vi "Add Item.vi"(7 "Action":T1, 8 "error in (no error)":errorcluster, 11 "Listbox Refs in":T2 {"Section Ref" format="%.0x"}) -> (0 "error out":errorcluster, 3 "Listbox Refs out":T2 {"Section Ref" format="%.0x"})   [LabVIEW 2015, in "FPGA Addon System Explorer.lvlib"]
uses:
  FPGA Addon System Explorer.lvlib
  Listbox Cluster.ctl
  <vilib>/NI Veristand/Custom Device API/Custom Device Item Ref.ctl
  Channel Type.ctl
  Shared/FG Action.ctl
  <vilib>/NI Veristand/Custom Device API/Custom Device Channel.ctl
  <vilib>/NI Veristand/Custom Device API/Custom Device Channel Type.ctl
  SubModules/FPGA Addon Speciality IO/Source/Types/PWM.Measure.Analog.Settings.ctl
  SubModules/FPGA Addon Speciality IO/Source/Types/PWM.Generate.Digital.Settings.ctl
  SubModules/FPGA Addon Speciality IO/Source/Types/PWM.Generate.Digital.Convert.Settings.ctl
  SubModules/FPGA Addon Speciality IO/Source/Types/WSS.Generate.Digital.Settings.ctl
  SubModules/FPGA Addon Speciality IO/Source/Types/WSS.Generate.Digital.Convert.Settings.ctl
  SubModules/FPGA Addon Speciality IO/Source/Types/WSS.Sensor.Type.ctl
  SubModules/FPGA Addon Speciality IO/Source/Types/Static.Generate.Digital.Settings.ctl
  SubModules/FPGA Addon Speciality IO/Source/Types/Static.Measure.Digital.Settings.ctl
  SubModules/FPGA Addon Speciality IO/Source/Types/Sine.Generate.Settings.ctl
  SubModules/FPGA Addon Speciality IO/Source/Types/Sine.Generate.Convert.Settings.ctl
  SubModules/FPGA Addon Speciality IO/Source/Types/PWM.Measure.Digital.Settings.ctl
  SubModules/FPGA Addon Speciality IO/Source/Types/PWM.Measure.Analog.Result.ctl
  SubModules/FPGA Addon Speciality IO/Source/Types/PWM.Measure.Digital.Result.ctl
  SubModules/FPGA Addon Speciality IO/Source/Types/Static.Measure.Digital.Measurement.ctl
  Shared/Constants.vi
  <vilib>/NI Veristand/Custom Device API/NI VeriStand - Set Item Property.vi
  <vilib>/NI Veristand/Custom Device API/Set Item Property (Variant).vi
  <vilib>/NI Veristand/Custom Device API/NI VeriStand - Get Item Property.vi
  <vilib>/NI Veristand/Custom Device API/Get Item Property (Variant).vi
  <vilib>/NI VeriStand/Custom Device API/Custom Device API.lvlib
  Shared/FPGA Addon Shared.lvlib
  SubModules/FPGA Addon Speciality IO/Source/Speciality FPGA IO.lvlib
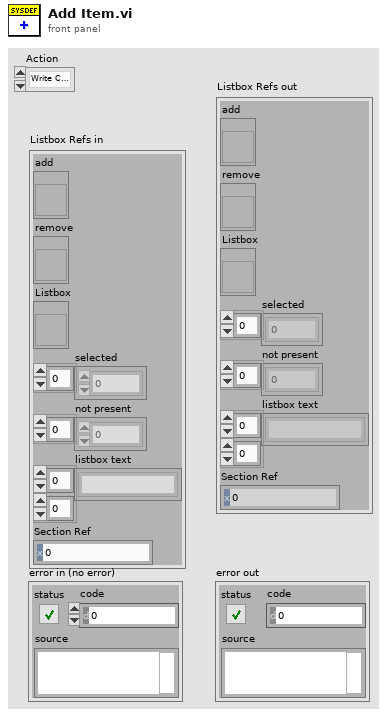
[diagram p1: front panel]
types:
  T1 = typedef "FPGA Addon System Explorer.lvlib/Channel Type.ctl" = enum16{"Write Channel", "Read Channel", "Write Waveform", "Read Waveform"}
  T2 = typedef "FPGA Addon System Explorer.lvlib/Listbox Cluster.ctl" = cluster{"add":refnum<vi>, "remove":refnum<vi>, "Listbox":refnum<vi>, "selected":i32[], "not present":i32[], "listbox text":string[][], "Section Ref":T3}
  T3 = typedef "Custom Device API.lvlib/Custom Device Item Ref.ctl" = u64
  T4 = typedef "Custom Device API.lvlib/Custom Device Channel.ctl" = cluster{"Type":T5, "Units":string, "Default Value":dbl, "Faultable":bool, "Scalable":bool}
  T5 = typedef "Custom Device API.lvlib/Custom Device Channel Type.ctl" = enum16{"Input", "Output"}
  T6 = typedef "FPGA Addon Shared.lvlib/FG Action.ctl" = enum8{"GET", "SET"}
  T7 = typedef "Speciality FPGA IO.lvlib/PWM.Measure.Analog.Settings.ctl" = cluster{"ACTIVE EDGE":bool, "TIMEOUT":u32, "THRESHOLD":fxp<+/-,32,8>}
  T8 = typedef "Speciality FPGA IO.lvlib/PWM.Generate.Digital.Convert.Settings.ctl" = cluster{"ACTIVE EDGE":bool, "FREQ":sgl, "DC":sgl}
  T9 = typedef "Speciality FPGA IO.lvlib/PWM.Generate.Digital.Settings.ctl" = cluster{"ACTIVE EDGE":bool, "ACTIVE TICKS":u32, "INACTIVE TICKS":u32}
  T10 = typedef "Speciality FPGA IO.lvlib/WSS.Generate.Digital.Convert.Settings.ctl" = cluster{"SPEED":u32, "DATA":u8, "PPR":u32, "WD":u32, "TYPE":u8}
  T11 = typedef "Speciality FPGA IO.lvlib/WSS.Generate.Digital.Settings.ctl" = cluster{"ACTIVE EDGE":bool, "ACTIVE TICKS":u32, "INACTIVE TICKS":u32, "DATA":u8, "SENSOR TYPE":u8}
  T12 = typedef "Speciality FPGA IO.lvlib/WSS.Sensor.Type.ctl" = enum16{"Unidirectional", "Bosch Bidirectional", "Continental Bidirectional"}
  T13 = typedef "Speciality FPGA IO.lvlib/Sine.Generate.Convert.Settings.ctl" = cluster{"AMP":sgl, "OFFSET":sgl, "FREQ":sgl}
  T14 = typedef "Speciality FPGA IO.lvlib/Sine.Generate.Settings.ctl" = cluster{"AMP":fxp<+/-,32,8>, "OFFSET":fxp<+/-,32,8>, "PERIODS/TICKS":fxp<+,32,0>}
  T15 = typedef "Speciality FPGA IO.lvlib/PWM.Measure.Analog.Result.ctl" = cluster{"FREQ":sgl, "PERIOD":sgl, "DC":sgl, "ACTIVE TIME":sgl, "ACTIVE VOLTAGE":sgl, "INACTIVE VOLTAGE":sgl}
  T16 = typedef "Speciality FPGA IO.lvlib/PWM.Measure.Digital.Result.ctl" = cluster{"FREQ":sgl, "PERIOD":sgl, "DC":sgl, "ACTIVE TIME":sgl}
  T17 = typedef "Speciality FPGA IO.lvlib/Static.Measure.Digital.Measurement.ctl" = cluster{"STATE":bool}
  T18 = typedef "FPGA Addon Shared.lvlib/Register Information.ctl" = cluster{"Name":string, "Data Type":T19, "Default Value":variant}
  T19 = typedef "FPGA Addon Shared.lvlib/Data Type.ctl" = enum8{"<Null>", "I8", "I16", "I32", "I64", "U8", "U16", "U32", "U64", "SGL", "Boolean", "Analog PWM In Settings", "Analog PWM In", "Digital PWM In Settings", "Digital PWM In", "Digital PWM Out", "Sine Out", "FXP+/-24.5", "FXP+/-16.5", "FXP+/-32.8", "FXP+/-64.32", "FXP+/-16.7", "FXP+/-20.5", "FXP+/-27.5", "FXP+/-32.16", "Digital Static In", "Digital Static Out", "Digital Static In Settings", "Digital WSS Out"}
  T20 = typedef "Speciality FPGA IO.lvlib/Static.Generate.Digital.Settings.ctl" = cluster{"ACTIVE EDGE":bool, "OUTPUT":bool}
  T21 = typedef "Speciality FPGA IO.lvlib/Static.Measure.Digital.Settings.ctl" = cluster{"ACTIVE EDGE":bool}
  T22 = typedef "Speciality FPGA IO.lvlib/PWM.Measure.Digital.Settings.ctl" = cluster{"ACTIVE EDGE":bool, "TIMEOUT":u32}
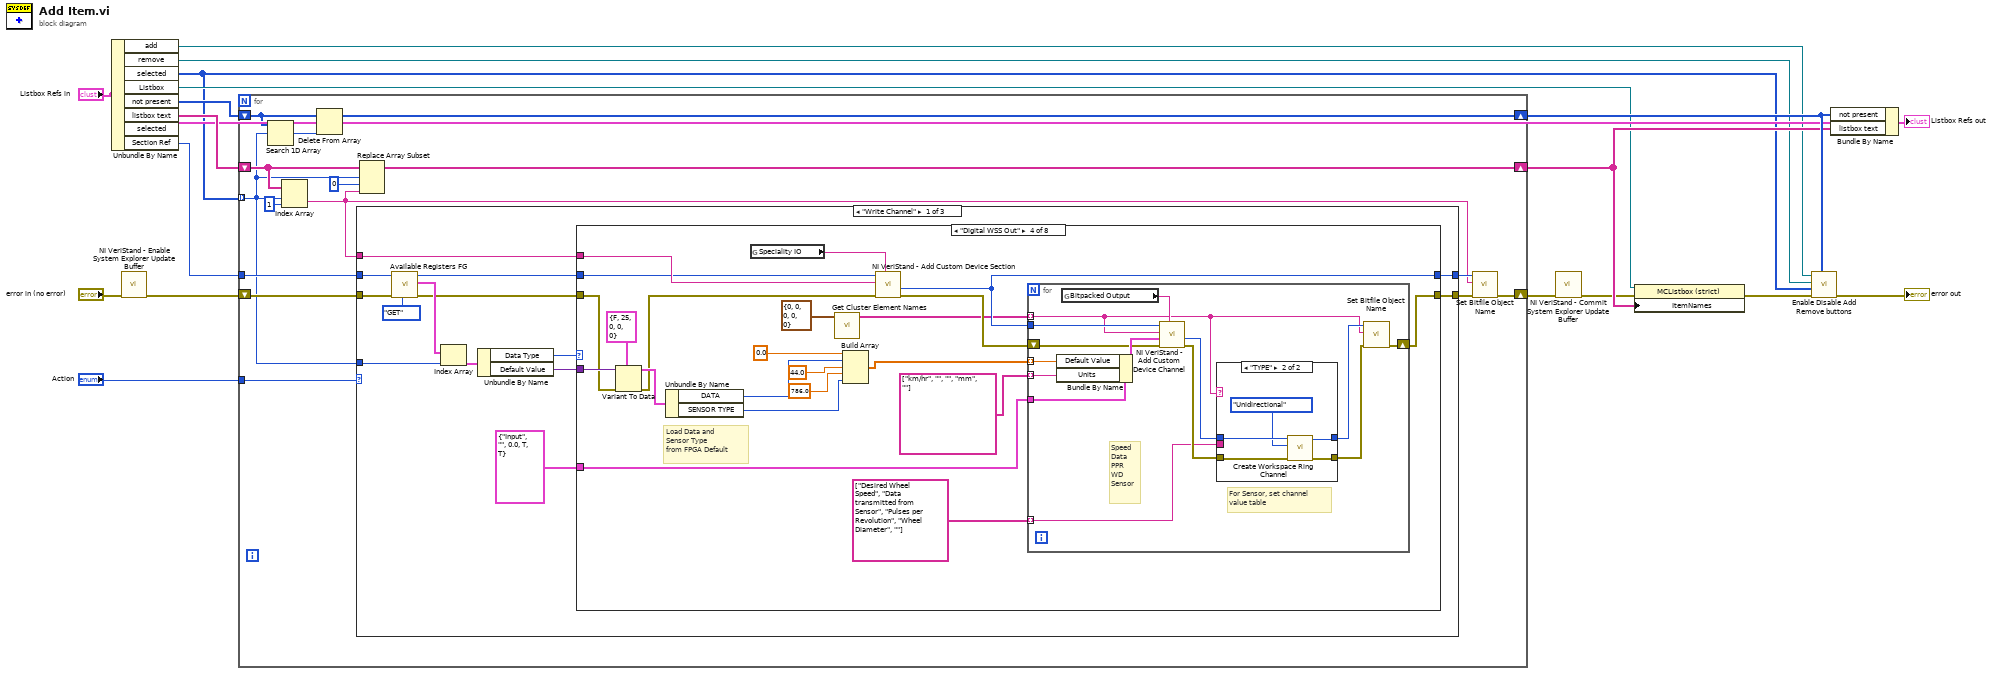
[diagram p0: block diagram]
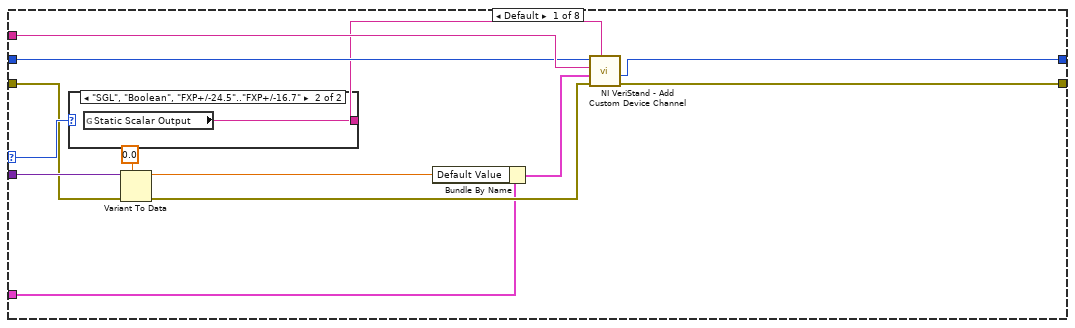
[diagram p2: hidden frame]
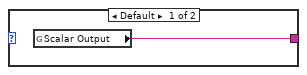
[diagram p3: hidden frame]
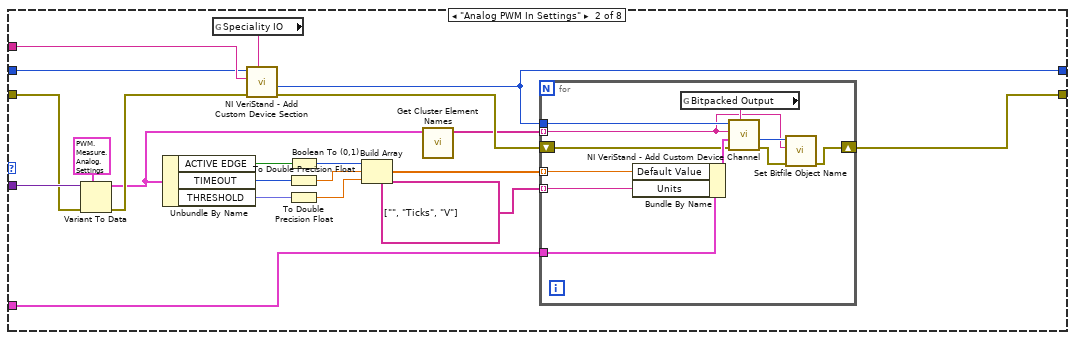
[diagram p4: hidden frame]
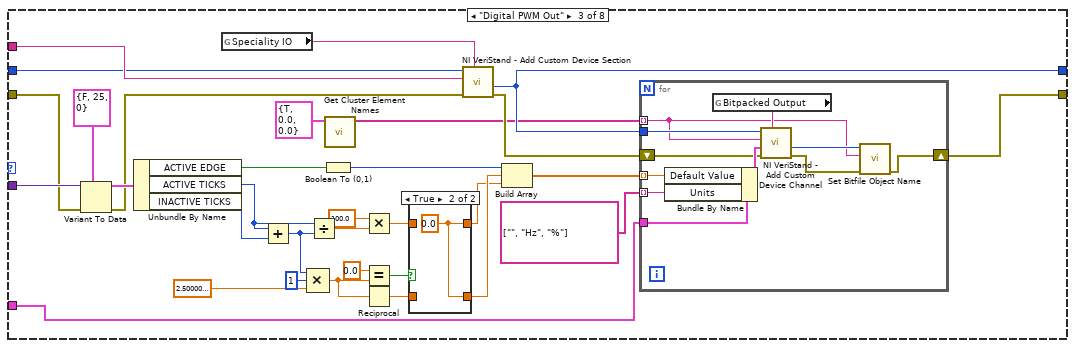
[diagram p5: hidden frame]
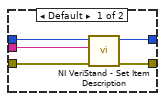
[diagram p7: hidden frame]
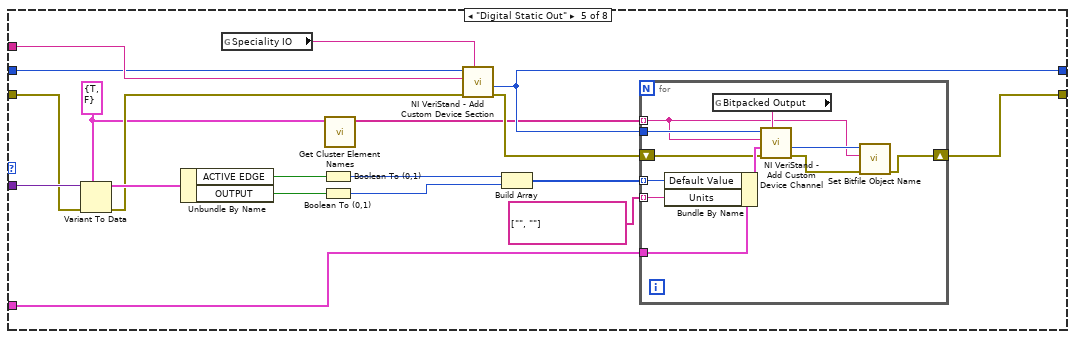
[diagram p8: hidden frame]
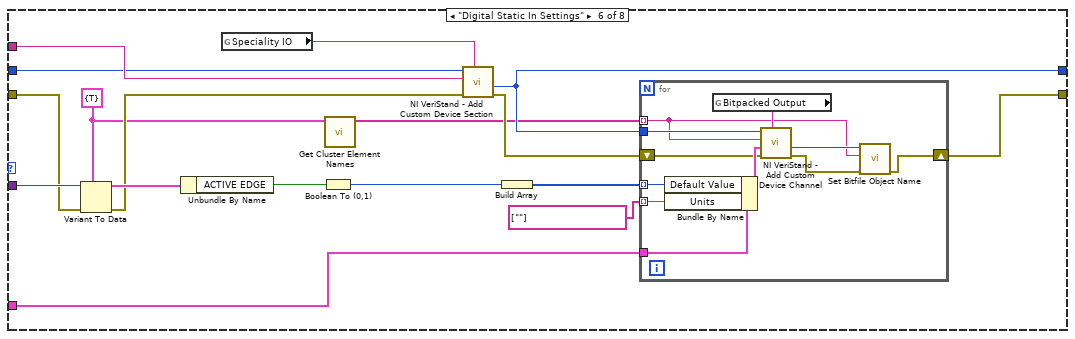
[diagram p9: hidden frame]
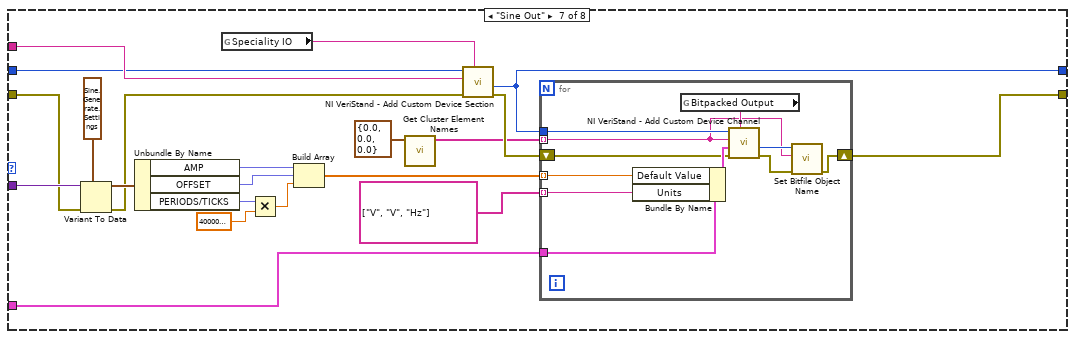
[diagram p10: hidden frame]
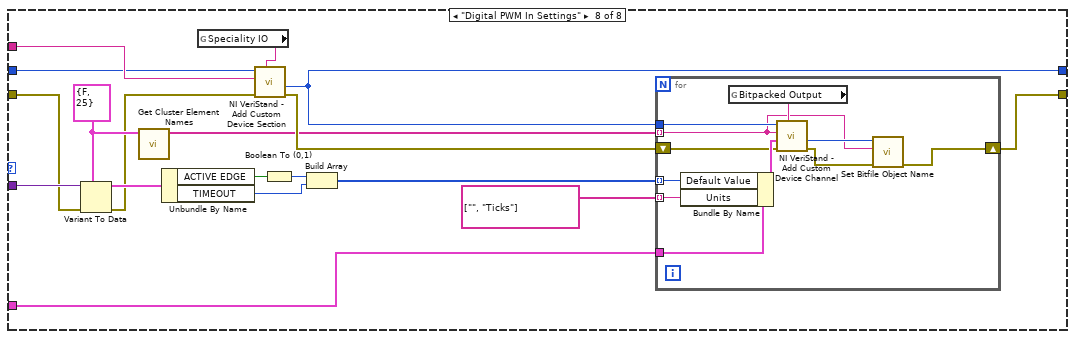
[diagram p11: hidden frame]
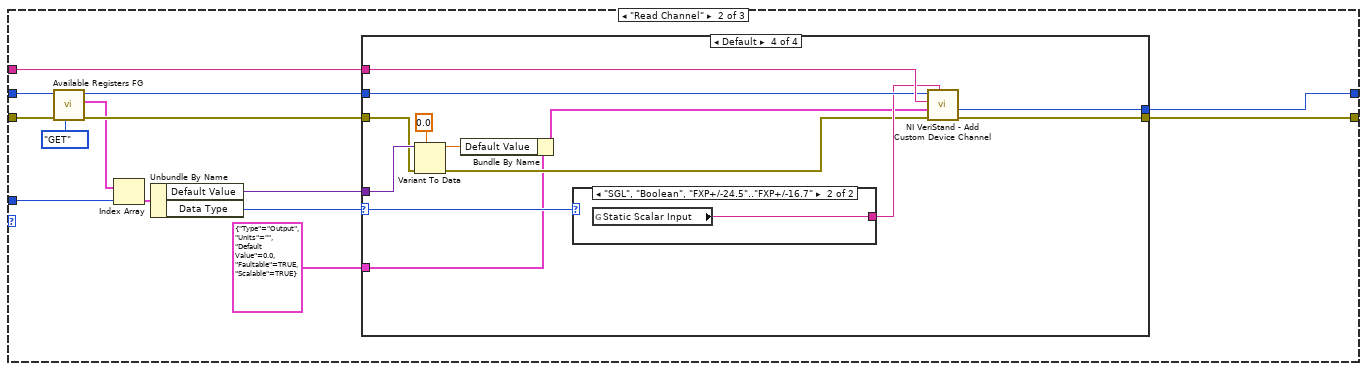
[diagram p12: hidden frame]
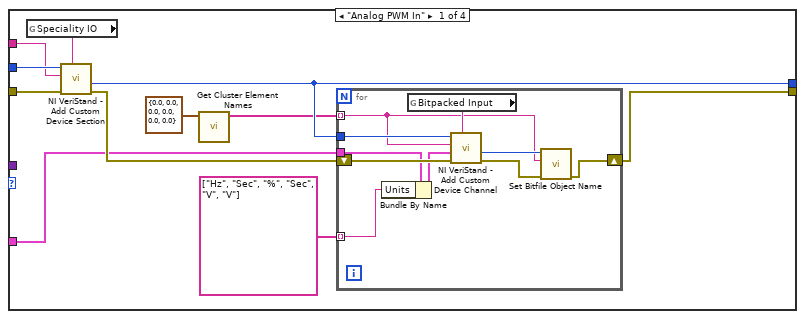
[diagram p13: hidden frame]
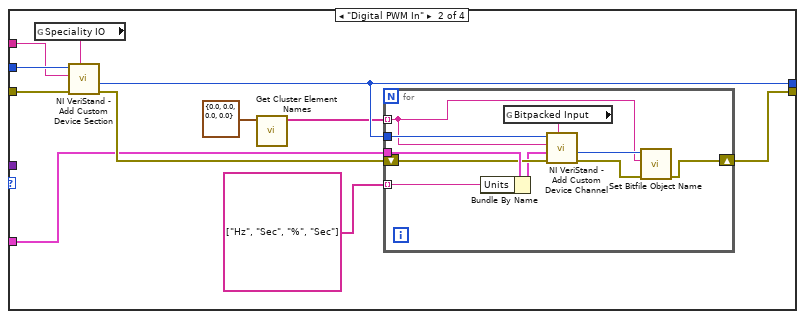
[diagram p14: hidden frame]
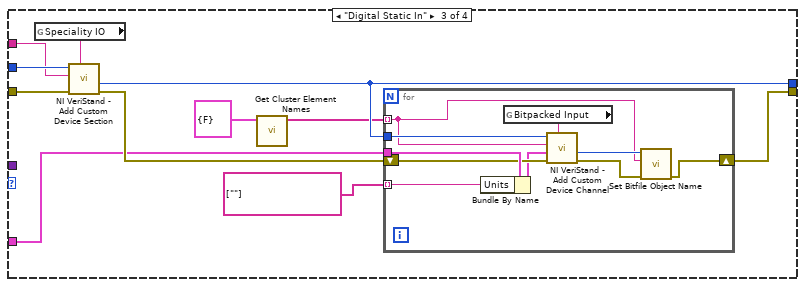
[diagram p15: hidden frame]
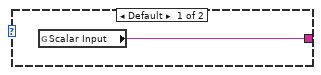
[diagram p16: hidden frame]
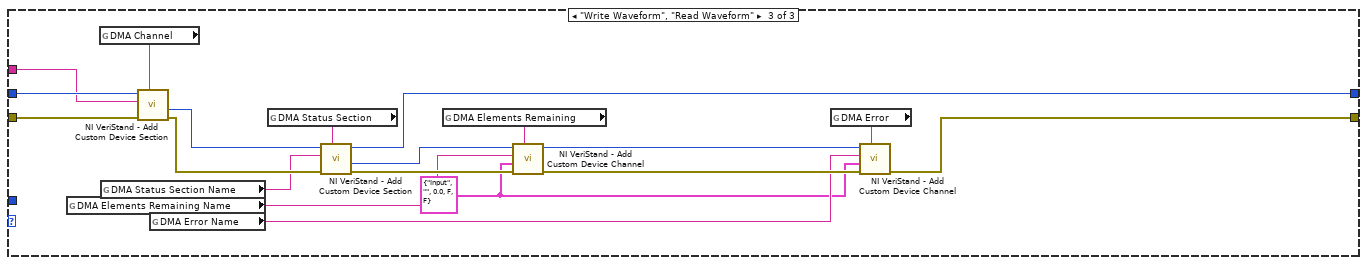
[diagram p17: hidden frame]
diagram:
  n1 = Unbundle By Name("Listbox Refs in") -> ("add"=w10:refnum<vi>, "remove"=w11:refnum<vi>, "selected"=w3:i32[], "Listbox"=w4:refnum<vi>, "not present"=w9:i32[], "listbox text"=w17:string[][], "Section Ref"=w5:T3)  [unwired: 1 out]
  n2 = call <vilib>:"NI VeriStand - Enable System Explorer Update Buffer.vi"("error in (no error)"="error in (no error)") -> ("error out"=w8:errorcluster)  [unwired: 10 in]
  n3 = for {
    tunnel: w5 -> [w32]
    shift-right: [w19] -> w6
    shift-left: w8 -> [w33]
    tunnel: w3 -> [w23] mode=indexing
    shift-right: [w29] -> w15
    shift-left: w17 -> [w30]
    shift-right: [w25] -> w16
    shift-left: w9 -> [w27]
    tunnel: "Action" -> [w24]
    n4 = Search 1D Array(1D array=w27, element=w23) -> (index of element=w26:i32)  [unwired: 1 in]
    n5 = Index Array(array=w30, index (row)=w23, index (col)=1 ("disabled index (col)")) -> (element=w21:string)
    n6 = Delete From Array(array=w27, index=w26) -> (array with subset deleted=w25:i32[])  [unwired: 1 in, 1 out]
    n7 = case shown="\"Write Channel\"" w24 {
      tunnel: w33 -> [w41 w314 w415]
      tunnel: [w47 w319 w406] -> w20
      tunnel: w32 -> [w40 w315 w416]
      tunnel: w21 -> [w46 w318 w400]
      tunnel: [w45 w317 w411] -> w22
      tunnel: w23 -> [w37 w310 _]
      frame "Write Channel" {
        n8 = call "Available Registers FG.vi"("Action"=FG_Action."GET", "error in (no error)"=w41, "Item Ref"=w40) -> ("error out"=w38:errorcluster, "Available Registers"=w43:T18[], "Item Ref out"=w39:T3)  [unwired: 6 in]
        n9 = Index Array(array=w43, index=w37) -> (element=w42:T18)
        n10 = Unbundle By Name(w42) -> ("Data Type"=w35:T19, "Default Value"=w36:variant)
        n11 = case shown="\"Digital WSS Out\"" w35 {
          selector: w35 -> [w54 _ _ _ _ _ _ _]
          tunnel: [w60 w77 w120 w156 w199 w227 w259 w288] -> w47
          tunnel: w46 -> [w59 w83 w126 w162 w205 w233 w265 w294]
          tunnel: [w58 w76 w122 w158 w201 w229 w261 w290] -> w45
          tunnel: w39 -> [w57 w82 w125 w161 w204 w232 w264 w293]
          tunnel: w38 -> [w50 w80 w123 w159 w202 w230 w262 w291]
          tunnel: w36 -> [w53 w81 w124 w160 w203 w231 w263 w292]
          tunnel: T4 {"Type"=enum."Input", "Units"="", "Default Value"=0.0, "Faultable"=TRUE, "Scalable"=TRUE} ("Channel") -> [w48 w63 w95 w147 w187 w217 w245 w277]
          frame Default {
            n12 = case shown="\"SGL\", \"Boolean\", \"FXP+/-24.5\"..\"FXP+/-16.7\"" w54 {
              tunnel: [w61 w62] -> w56
              frame Default {
                n13 = global read "Constants.vi" "Scalar Output"() -> (w61:string)
              }
              frame "SGL", "Boolean", "FXP+/-24.5".."FXP+/-16.7" {
                n14 = global read "Constants.vi" "Static Scalar Output"() -> (w62:string)
              }
            }
            n15 = Variant To Data(error in=w50, type=0.0 ("Default Value"), Variant=w53) -> (data=w51:dbl, error out=w49:errorcluster)
            n16 = Bundle By Name(cluster=w48, "Default Value"=w51) -> (w55:T4)
            n17 = call <vilib>:"NI VeriStand - Add Custom Device Channel.vi"("GUID (Default Channel)"=w56, "error in (no error)"=w49, "Channel"=w55, "Channel Name"=w59, "Parent Ref in"=w57) -> ("error out"=w60:errorcluster, "Channel Ref"=w58:T3)  [unwired: 3 in, 2 out]
          }
          frame "Analog PWM In Settings" {
            n18 = Variant To Data(error in=w80, type=T7 {"ACTIVE EDGE"=FALSE, "TIMEOUT"=1000000000, "THRESHOLD"=25.0} ("Channel.Settings"), Variant=w81) -> (data=w65:T7, error out=w66:errorcluster)
            n19 = Unbundle By Name(w65) -> ("ACTIVE EDGE"=w71:bool, "TIMEOUT"=w75:u32, "THRESHOLD"=w70:fxp<+/-,32,8>)
            n20 = global read "Constants.vi" "Speciality IO"() -> (w67:string)
            n21 = call <vilib>:"NI VeriStand - Add Custom Device Section.vi"("GUID (Default Section)"=w67, "error in (no error)"=w66, "Section Name"=w83, "Parent Ref in"=w82) -> ("error out"=w78:errorcluster, "Section Ptr"=w76:T3)  [unwired: 4 in, 2 out]
            n22 = Boolean To (0,1)(Boolean=w71) -> (0, 1=w69:i16)
            n23 = To Double Precision Float(number=w75) -> (double precision float=w73:dbl)
            n24 = To Double Precision Float(number=w70) -> (double precision float=w68:dbl)
            n25 = Build Array(w69, w73, w68) -> (w74:dbl[])
            n26 = call "Get Cluster Element Names.vi"("Cluster"=w65) -> ("Channels"=w64:string[])  [unwired: 10 in]
            n27 = for {
              tunnel: w76 -> [w93]
              shift-right: [w86] -> w77
              shift-left: w78 -> [w92]
              tunnel: w74 -> [w90] mode=indexing
              tunnel: string[] ["", "Ticks", "V"] -> [w89] mode=indexing
              tunnel: w64 -> [w85] mode=indexing
              tunnel: w63 -> [w84]
              n28 = Bundle By Name(cluster=w84, "Default Value"=w90, "Units"=w89) -> (w94:T4)
              n29 = global read "Constants.vi" "Bitpacked Output"() -> (w91:string)
              n30 = call <vilib>:"NI VeriStand - Add Custom Device Channel.vi"("GUID (Default Channel)"=w91, "error in (no error)"=w92, "Channel"=w94, "Channel Name"=w85, "Parent Ref in"=w93) -> ("error out"=w87:errorcluster, "Channel Ref"=w88:T3)  [unwired: 3 in, 2 out]
              n31 = call "Set Bitfile Object Name.vi"("error in (no error)"=w87, "Name"=w85, "Channel Ref"=w88) -> ("error out"=w86:errorcluster)  [unwired: 8 in]
            }
          }
          frame "Digital PWM Out" {
            n32 = Variant To Data(error in=w123, type=T9 {"ACTIVE EDGE"=FALSE, "ACTIVE TICKS"=25, "INACTIVE TICKS"=0} ("Channel.Settings"), Variant=w124) -> (data=w119:T9, error out=w112:errorcluster)
            n33 = Unbundle By Name(w119) -> ("ACTIVE EDGE"=w118:bool, "ACTIVE TICKS"=w103:u32, "INACTIVE TICKS"=w102:u32)
            n34 = global read "Constants.vi" "Speciality IO"() -> (w115:string)
            n35 = Add(x=w103, y=w102) -> (x+y=w109:u32)
            n36 = Compound Arithmetic op=MULTIPLY(w109, u32 1 ("value"), 2.5000000292152436e-08 ("y")) -> (w110:dbl)
            n37 = Divide(x=w103, y=w109) -> (x/y=w105:dbl)
            n38 = Boolean To (0,1)(Boolean=w118) -> (0, 1=w117:i16)
            n39 = call "Get Cluster Element Names.vi"("Cluster"=T8 {"ACTIVE EDGE"=TRUE, "FREQ"=0.0, "DC"=0.0} ("Settings")) -> ("Channels"=w113:string[])  [unwired: 10 in]
            n40 = Multiply(x=100.0, y=w105) -> (x*y=w97:dbl)
            n41 = Equal?(x=0.0, y=w110) -> (x = y?=w101:bool)
            n42 = Reciprocal(x=w110) -> (1/x=w99:dbl)
            n43 = case shown="True" w101 {
              tunnel: [w128 w129] -> w100
              tunnel: w99 -> [w128 _]
              tunnel: [w127 w129] -> w98
              tunnel: w97 -> [w127 _]
              frame False {
              }
              frame True {
                w129 = 0.0
              }
            }
            n44 = call <vilib>:"NI VeriStand - Add Custom Device Section.vi"("GUID (Default Section)"=w115, "error in (no error)"=w112, "Section Name"=w126, "Parent Ref in"=w125) -> ("error out"=w121:errorcluster, "Section Ptr"=w122:T3)  [unwired: 4 in, 2 out]
            n45 = Build Array(w117, w100, w98) -> (w116:dbl[])
            n46 = for {
              tunnel: w122 -> [w139]
              shift-right: [w132] -> w120
              shift-left: w121 -> [w138]
              tunnel: w116 -> [w136] mode=indexing
              tunnel: w113 -> [w131] mode=indexing
              tunnel: string[] ["", "Hz", "%"] -> [w135] mode=indexing
              tunnel: w95 -> [w130]
              n47 = Bundle By Name(cluster=w130, "Default Value"=w136, "Units"=w135) -> (w140:T4)
              n48 = global read "Constants.vi" "Bitpacked Output"() -> (w137:string)
              n49 = call <vilib>:"NI VeriStand - Add Custom Device Channel.vi"("GUID (Default Channel)"=w137, "error in (no error)"=w138, "Channel"=w140, "Channel Name"=w131, "Parent Ref in"=w139) -> ("error out"=w133:errorcluster, "Channel Ref"=w134:T3)  [unwired: 3 in, 2 out]
              n50 = call "Set Bitfile Object Name.vi"("error in (no error)"=w133, "Name"=w131, "Channel Ref"=w134) -> ("error out"=w132:errorcluster)  [unwired: 8 in]
            }
          }
          frame "Digital WSS Out" {
            # "Load Data and\nSensor Type\nfrom FPGA Default"
            n51 = Variant To Data(error in=w159, type=T11 {"ACTIVE EDGE"=FALSE, "ACTIVE TICKS"=25, "INACTIVE TICKS"=0, "DATA"=0, "SENSOR TYPE"=0} ("Channel.Settings"), Variant=w160) -> (data=w155:T11, error out=w150:errorcluster)
            n52 = Unbundle By Name(w155) -> ("DATA"=w141:u8, "SENSOR TYPE"=w142:u8)
            n53 = global read "Constants.vi" "Speciality IO"() -> (w153:string)
            n54 = call "Get Cluster Element Names.vi"("Cluster"=T10 {"SPEED"=0, "DATA"=0, "PPR"=0, "WD"=0, "TYPE"=0} ("Wheel Speed Sensor Settings")) -> ("Channels"=w151:string[])  [unwired: 10 in]
            n55 = Build Array(0.0 ("element"), w141, 44.0 ("element"), 786.0 ("element"), w142) -> (w154:dbl[])
            n56 = call <vilib>:"NI VeriStand - Add Custom Device Section.vi"("GUID (Default Section)"=w153, "error in (no error)"=w150, "Section Name"=w162, "Parent Ref in"=w161) -> ("error out"=w157:errorcluster, "Section Ptr"=w158:T3)  [unwired: 4 in, 2 out]
            n57 = for {
              tunnel: w158 -> [w175]
              shift-right: [w170] -> w156
              shift-left: w157 -> [w174]
              tunnel: w154 -> [w172] mode=indexing
              tunnel: w151 -> [w163] mode=indexing
              tunnel: string[] ["km/hr", "", "", "mm", ""] -> [w171] mode=indexing
              tunnel: w147 -> [w169]
              tunnel: string[] ["Desired Wheel Speed", "Data transmitted from Sensor", "Pulses per Revolution", "Wheel Diameter", ""] -> [w164] mode=indexing
              # "For Sensor, set channel \nvalue table"
              # "Speed\nData\nPPR\nWD\nSensor"
              n58 = Bundle By Name(cluster=w169, "Default Value"=w172, "Units"=w171) -> (w176:T4)
              n59 = global read "Constants.vi" "Bitpacked Output"() -> (w173:string)
              n60 = call <vilib>:"NI VeriStand - Add Custom Device Channel.vi"("GUID (Default Channel)"=w173, "error in (no error)"=w174, "Channel"=w176, "Channel Name"=w163, "Parent Ref in"=w175) -> ("error out"=w168:errorcluster, "Channel Ref"=w166:T3)  [unwired: 3 in, 2 out]
              n61 = case shown="\"TYPE\"" w163 {
                tunnel: w168 -> [w181 w185]
                tunnel: [w180 w184] -> w167
                tunnel: w166 -> [w179 w186]
                tunnel: [w178 w183] -> w165
                tunnel: w164 -> [w177 _]
                frame Default {
                  n62 = call <vilib>:"NI VeriStand - Set Item Description.vi"("error in (no error)"=w181, "Description"=w177, "Item Ref in"=w179) -> ("error out"=w180:errorcluster, "Item Ref out"=w178:T3)  [unwired: 6 in, 1 out]
                }
                frame "TYPE" {
                  n63 = call "Create Workspace Ring Channel.vi"("error in (no error)"=w185, "Enum"=WSS.Sensor.Type."Unidirectional" ("Sensor Type"), "Channel Ref in"=w186) -> ("error out"=w184:errorcluster, "Channel Ref out"=w183:T3)  [unwired: 7 in]
                }
              }
              n64 = call "Set Bitfile Object Name.vi"("error in (no error)"=w167, "Name"=w163, "Channel Ref"=w165) -> ("error out"=w170:errorcluster)  [unwired: 8 in]
            }
          }
          frame "Digital Static Out" {
            w190 = T20 {"ACTIVE EDGE"=TRUE, "OUTPUT"=FALSE} ("Settings")
            n65 = Variant To Data(error in=w202, type=w190, Variant=w203) -> (data=w198:T20, error out=w192:errorcluster)
            n66 = Unbundle By Name(w198) -> ("ACTIVE EDGE"=w197:bool, "OUTPUT"=w189:bool)
            n67 = global read "Constants.vi" "Speciality IO"() -> (w194:string)
            n68 = Boolean To (0,1)(Boolean=w197) -> (0, 1=w196:i16)
            n69 = Boolean To (0,1)(Boolean=w189) -> (0, 1=w188:i16)
            n70 = call "Get Cluster Element Names.vi"("Cluster"=w190) -> ("Channels"=w193:string[])  [unwired: 10 in]
            n71 = call <vilib>:"NI VeriStand - Add Custom Device Section.vi"("GUID (Default Section)"=w194, "error in (no error)"=w192, "Section Name"=w205, "Parent Ref in"=w204) -> ("error out"=w200:errorcluster, "Section Ptr"=w201:T3)  [unwired: 4 in, 2 out]
            n72 = Build Array(w196, w188) -> (w195:i16[])
            n73 = for {
              tunnel: w201 -> [w215]
              shift-right: [w208] -> w199
              shift-left: w200 -> [w214]
              tunnel: w195 -> [w212] mode=indexing
              tunnel: w193 -> [w207] mode=indexing
              tunnel: string[] ["", ""] -> [w211] mode=indexing
              tunnel: w187 -> [w206]
              n74 = Bundle By Name(cluster=w206, "Default Value"=w212, "Units"=w211) -> (w216:T4)
              n75 = global read "Constants.vi" "Bitpacked Output"() -> (w213:string)
              n76 = call <vilib>:"NI VeriStand - Add Custom Device Channel.vi"("GUID (Default Channel)"=w213, "error in (no error)"=w214, "Channel"=w216, "Channel Name"=w207, "Parent Ref in"=w215) -> ("error out"=w209:errorcluster, "Channel Ref"=w210:T3)  [unwired: 3 in, 2 out]
              n77 = call "Set Bitfile Object Name.vi"("error in (no error)"=w209, "Name"=w207, "Channel Ref"=w210) -> ("error out"=w208:errorcluster)  [unwired: 8 in]
            }
          }
          frame "Digital Static In Settings" {
            w218 = T21 {"ACTIVE EDGE"=TRUE} ("Settings")
            n78 = Variant To Data(error in=w230, type=w218, Variant=w231) -> (data=w226:T21, error out=w220:errorcluster)
            n79 = Unbundle By Name(w226) -> ("ACTIVE EDGE"=w225:bool)
            n80 = global read "Constants.vi" "Speciality IO"() -> (w222:string)
            n81 = Boolean To (0,1)(Boolean=w225) -> (0, 1=w224:i16)
            n82 = call "Get Cluster Element Names.vi"("Cluster"=w218) -> ("Channels"=w221:string[])  [unwired: 10 in]
            n83 = call <vilib>:"NI VeriStand - Add Custom Device Section.vi"("GUID (Default Section)"=w222, "error in (no error)"=w220, "Section Name"=w233, "Parent Ref in"=w232) -> ("error out"=w228:errorcluster, "Section Ptr"=w229:T3)  [unwired: 4 in, 2 out]
            n84 = Build Array(w224) -> (w223:i16[])
            n85 = for {
              tunnel: w229 -> [w243]
              shift-right: [w236] -> w227
              shift-left: w228 -> [w242]
              tunnel: w223 -> [w240] mode=indexing
              tunnel: w221 -> [w235] mode=indexing
              tunnel: string[] [""] -> [w239] mode=indexing
              tunnel: w217 -> [w234]
              n86 = Bundle By Name(cluster=w234, "Default Value"=w240, "Units"=w239) -> (w244:T4)
              n87 = global read "Constants.vi" "Bitpacked Output"() -> (w241:string)
              n88 = call <vilib>:"NI VeriStand - Add Custom Device Channel.vi"("GUID (Default Channel)"=w241, "error in (no error)"=w242, "Channel"=w244, "Channel Name"=w235, "Parent Ref in"=w243) -> ("error out"=w237:errorcluster, "Channel Ref"=w238:T3)  [unwired: 3 in, 2 out]
              n89 = call "Set Bitfile Object Name.vi"("error in (no error)"=w237, "Name"=w235, "Channel Ref"=w238) -> ("error out"=w236:errorcluster)  [unwired: 8 in]
            }
          }
          frame "Sine Out" {
            n90 = Variant To Data(error in=w262, type=T14 {"AMP"=0.0, "OFFSET"=0.0, "PERIODS/TICKS"=0.0} ("Settings"), Variant=w263) -> (data=w258:T14, error out=w253:errorcluster)
            n91 = Unbundle By Name(w258) -> ("AMP"=w251:fxp<+/-,32,8>, "OFFSET"=w250:fxp<+/-,32,8>, "PERIODS/TICKS"=w249:fxp<+,32,0>)
            n92 = global read "Constants.vi" "Speciality IO"() -> (w256:string)
            n93 = Multiply(x=w249, y=sgl 40000000.0) -> (x*y=w247:sgl)
            n94 = Build Array(w251, w250, w247) -> (w257:sgl[])
            n95 = call "Get Cluster Element Names.vi"("Cluster"=T13 {"AMP"=0.0, "OFFSET"=0.0, "FREQ"=0.0} ("Settings")) -> ("Channels"=w254:string[])  [unwired: 10 in]
            n96 = call <vilib>:"NI VeriStand - Add Custom Device Section.vi"("GUID (Default Section)"=w256, "error in (no error)"=w253, "Section Name"=w265, "Parent Ref in"=w264) -> ("error out"=w260:errorcluster, "Section Ptr"=w261:T3)  [unwired: 4 in, 2 out]
            n97 = for {
              tunnel: w261 -> [w275]
              shift-right: [w268] -> w259
              shift-left: w260 -> [w274]
              tunnel: w257 -> [w272] mode=indexing
              tunnel: w254 -> [w267] mode=indexing
              tunnel: string[] ["V", "V", "Hz"] -> [w271] mode=indexing
              tunnel: w245 -> [w266]
              n98 = Bundle By Name(cluster=w266, "Default Value"=w272, "Units"=w271) -> (w276:T4)
              n99 = global read "Constants.vi" "Bitpacked Output"() -> (w273:string)
              n100 = call <vilib>:"NI VeriStand - Add Custom Device Channel.vi"("GUID (Default Channel)"=w273, "error in (no error)"=w274, "Channel"=w276, "Channel Name"=w267, "Parent Ref in"=w275) -> ("error out"=w269:errorcluster, "Channel Ref"=w270:T3)  [unwired: 3 in, 2 out]
              n101 = call "Set Bitfile Object Name.vi"("error in (no error)"=w269, "Name"=w267, "Channel Ref"=w270) -> ("error out"=w268:errorcluster)  [unwired: 8 in]
            }
          }
          frame "Digital PWM In Settings" {
            w281 = T22 {"ACTIVE EDGE"=FALSE, "TIMEOUT"=25} ("Channel.Settings")
            n102 = Variant To Data(error in=w291, type=w281, Variant=w292) -> (data=w284:T22, error out=w279:errorcluster)
            n103 = call "Get Cluster Element Names.vi"("Cluster"=w281) -> ("Channels"=w280:string[])  [unwired: 10 in]
            n104 = Unbundle By Name(w284) -> ("ACTIVE EDGE"=w287:bool, "TIMEOUT"=w286:u32)
            n105 = global read "Constants.vi" "Speciality IO"() -> (w282:string)
            n106 = call <vilib>:"NI VeriStand - Add Custom Device Section.vi"("GUID (Default Section)"=w282, "error in (no error)"=w279, "Section Name"=w294, "Parent Ref in"=w293) -> ("error out"=w289:errorcluster, "Section Ptr"=w290:T3)  [unwired: 4 in, 2 out]
            n107 = Boolean To (0,1)(Boolean=w287) -> (0, 1=w285:i16)
            n108 = Build Array(w285, w286) -> (w283:u32[])
            n109 = for {
              tunnel: w290 -> [w304]
              shift-right: [w298] -> w288
              shift-left: w289 -> [w303]
              tunnel: w283 -> [w301] mode=indexing
              tunnel: w280 -> [w296] mode=indexing
              tunnel: string[] ["", "Ticks"] -> [w300] mode=indexing
              tunnel: w277 -> [w295]
              n110 = Bundle By Name(cluster=w295, "Default Value"=w301, "Units"=w300) -> (w305:T4)
              n111 = global read "Constants.vi" "Bitpacked Output"() -> (w302:string)
              n112 = call <vilib>:"NI VeriStand - Add Custom Device Channel.vi"("GUID (Default Channel)"=w302, "error in (no error)"=w303, "Channel"=w305, "Channel Name"=w296, "Parent Ref in"=w304) -> ("error out"=w299:errorcluster, "Channel Ref"=w297:T3)  [unwired: 3 in, 2 out]
              n113 = call "Set Bitfile Object Name.vi"("error in (no error)"=w299, "Name"=w296, "Channel Ref"=w297) -> ("error out"=w298:errorcluster)  [unwired: 8 in]
            }
          }
        }
      }
      frame "Read Channel" {
        n114 = call "Available Registers FG.vi"("Action"=FG_Action."GET", "error in (no error)"=w314, "Item Ref"=w315) -> ("error out"=w313:errorcluster, "Available Registers"=w311:T18[], "Item Ref out"=w312:T3)  [unwired: 6 in]
        n115 = Index Array(array=w311, index=w310) -> (element=w309:T18)
        n116 = Unbundle By Name(w309) -> ("Default Value"=w307:variant, "Data Type"=w308:T19)
        n117 = case shown="Default" w308 {
          selector: w308 -> [_ _ _ w389]
          tunnel: [w326 w347 w368 w395] -> w319
          tunnel: w318 -> [w328 w349 w370 w394]
          tunnel: [w327 w348 w369 w393] -> w317
          tunnel: w313 -> [w330 w351 w372 w385]
          tunnel: w312 -> [w329 w350 w371 w392]
          tunnel: w307 -> [_ _ _ w388]
          tunnel: T4 {"Type"=enum."Output", "Units"="", "Default Value"=0.0, "Faultable"=TRUE, "Scalable"=TRUE} ("Channel") -> [w320 w341 w362 w383]
          frame "Analog PWM In" {
            n118 = global read "Constants.vi" "Speciality IO"() -> (w324:string)
            n119 = call <vilib>:"NI VeriStand - Add Custom Device Section.vi"("GUID (Default Section)"=w324, "error in (no error)"=w330, "Section Name"=w328, "Parent Ref in"=w329) -> ("error out"=w321:errorcluster, "Section Ptr"=w327:T3)  [unwired: 4 in, 2 out]
            n120 = call "Get Cluster Element Names.vi"("Cluster"=T15 {"FREQ"=0.0, "PERIOD"=0.0, "DC"=0.0, "ACTIVE TIME"=0.0, "ACTIVE VOLTAGE"=0.0, "INACTIVE VOLTAGE"=0.0} ("Analyzed")) -> ("Channels"=w322:string[])  [unwired: 10 in]
            n121 = for {
              tunnel: w320 -> [w337]
              tunnel: w327 -> [w340]
              shift-right: [w332] -> w326
              shift-left: w321 -> [w339]
              tunnel: string[] ["Hz", "Sec", "%", "Sec", "V", "V"] -> [w335] mode=indexing
              tunnel: w322 -> [w331] mode=indexing
              n122 = Bundle By Name(cluster=w337, "Units"=w335) -> (w336:T4)
              n123 = global read "Constants.vi" "Bitpacked Input"() -> (w338:string)
              n124 = call <vilib>:"NI VeriStand - Add Custom Device Channel.vi"("GUID (Default Channel)"=w338, "error in (no error)"=w339, "Channel"=w336, "Channel Name"=w331, "Parent Ref in"=w340) -> ("error out"=w333:errorcluster, "Channel Ref"=w334:T3)  [unwired: 3 in, 2 out]
              n125 = call "Set Bitfile Object Name.vi"("error in (no error)"=w333, "Name"=w331, "Channel Ref"=w334) -> ("error out"=w332:errorcluster)  [unwired: 8 in]
            }
          }
          frame "Digital PWM In" {
            n126 = global read "Constants.vi" "Speciality IO"() -> (w345:string)
            n127 = call <vilib>:"NI VeriStand - Add Custom Device Section.vi"("GUID (Default Section)"=w345, "error in (no error)"=w351, "Section Name"=w349, "Parent Ref in"=w350) -> ("error out"=w342:errorcluster, "Section Ptr"=w348:T3)  [unwired: 4 in, 2 out]
            n128 = call "Get Cluster Element Names.vi"("Cluster"=T16 {"FREQ"=0.0, "PERIOD"=0.0, "DC"=0.0, "ACTIVE TIME"=0.0} ("Analyzed")) -> ("Channels"=w343:string[])  [unwired: 10 in]
            n129 = for {
              tunnel: w341 -> [w361]
              tunnel: w348 -> [w360]
              shift-right: [w352] -> w347
              shift-left: w342 -> [w359]
              tunnel: string[] ["Hz", "Sec", "%", "Sec"] -> [w356] mode=indexing
              tunnel: w343 -> [w354] mode=indexing
              n130 = Bundle By Name(cluster=w361, "Units"=w356) -> (w357:T4)
              n131 = global read "Constants.vi" "Bitpacked Input"() -> (w358:string)
              n132 = call <vilib>:"NI VeriStand - Add Custom Device Channel.vi"("GUID (Default Channel)"=w358, "error in (no error)"=w359, "Channel"=w357, "Channel Name"=w354, "Parent Ref in"=w360) -> ("error out"=w353:errorcluster, "Channel Ref"=w355:T3)  [unwired: 3 in, 2 out]
              n133 = call "Set Bitfile Object Name.vi"("error in (no error)"=w353, "Name"=w354, "Channel Ref"=w355) -> ("error out"=w352:errorcluster)  [unwired: 8 in]
            }
          }
          frame "Digital Static In" {
            n134 = global read "Constants.vi" "Speciality IO"() -> (w366:string)
            n135 = call <vilib>:"NI VeriStand - Add Custom Device Section.vi"("GUID (Default Section)"=w366, "error in (no error)"=w372, "Section Name"=w370, "Parent Ref in"=w371) -> ("error out"=w363:errorcluster, "Section Ptr"=w369:T3)  [unwired: 4 in, 2 out]
            n136 = call "Get Cluster Element Names.vi"("Cluster"=T17 {"STATE"=FALSE} ("Analyzed")) -> ("Channels"=w364:string[])  [unwired: 10 in]
            n137 = for {
              tunnel: w362 -> [w382]
              tunnel: w369 -> [w381]
              shift-right: [w373] -> w368
              shift-left: w363 -> [w380]
              tunnel: string[] [""] -> [w377] mode=indexing
              tunnel: w364 -> [w375] mode=indexing
              n138 = Bundle By Name(cluster=w382, "Units"=w377) -> (w378:T4)
              n139 = global read "Constants.vi" "Bitpacked Input"() -> (w379:string)
              n140 = call <vilib>:"NI VeriStand - Add Custom Device Channel.vi"("GUID (Default Channel)"=w379, "error in (no error)"=w380, "Channel"=w378, "Channel Name"=w375, "Parent Ref in"=w381) -> ("error out"=w374:errorcluster, "Channel Ref"=w376:T3)  [unwired: 3 in, 2 out]
              n141 = call "Set Bitfile Object Name.vi"("error in (no error)"=w374, "Name"=w375, "Channel Ref"=w376) -> ("error out"=w373:errorcluster)  [unwired: 8 in]
            }
          }
          frame Default {
            n142 = Variant To Data(error in=w385, type=0.0, Variant=w388) -> (data=w386:dbl, error out=w384:errorcluster)
            n143 = Bundle By Name(cluster=w383, "Default Value"=w386) -> (w390:T4)
            n144 = case shown="\"SGL\", \"Boolean\", \"FXP+/-24.5\"..\"FXP+/-16.7\"" w389 {
              tunnel: [w396 w397] -> w391
              frame Default {
                n145 = global read "Constants.vi" "Scalar Input"() -> (w396:string)
              }
              frame "SGL", "Boolean", "FXP+/-24.5".."FXP+/-16.7" {
                n146 = global read "Constants.vi" "Static Scalar Input"() -> (w397:string)
              }
            }
            n147 = call <vilib>:"NI VeriStand - Add Custom Device Channel.vi"("GUID (Default Channel)"=w391, "error in (no error)"=w384, "Channel"=w390, "Channel Name"=w394, "Parent Ref in"=w392) -> ("error out"=w395:errorcluster, "Channel Ref"=w393:T3)  [unwired: 3 in, 2 out]
          }
        }
      }
      frame "Write Waveform", "Read Waveform" {
        w401 = T4 {"Type"=enum."Input", "Units"="", "Default Value"=0.0, "Faultable"=FALSE, "Scalable"=FALSE} ("Channel")
        n148 = global read "Constants.vi" "DMA Elements Remaining Name"() -> (w404:string)
        n149 = global read "Constants.vi" "DMA Channel"() -> (w414:string)
        n150 = global read "Constants.vi" "DMA Status Section Name"() -> (w399:string)
        n151 = call <vilib>:"NI VeriStand - Add Custom Device Section.vi"("GUID (Default Section)"=w414, "error in (no error)"=w415, "Section Name"=w400, "Parent Ref in"=w416) -> ("error out"=w413:errorcluster, "Section Ptr"=w412:T3)  [unwired: 4 in, 2 out]
        n152 = global read "Constants.vi" "DMA Error Name"() -> (w403:string)
        n153 = global read "Constants.vi" "DMA Status Section"() -> (w398:string)
        n154 = call <vilib>:"NI VeriStand - Add Custom Device Section.vi"("GUID (Default Section)"=w398, "error in (no error)"=w413, "Section Name"=w399, "Parent Ref in"=w412) -> ("error out"=w407:errorcluster, "Section Ptr"=w408:T3, "Parent Ref out"=w411:T3)  [unwired: 4 in, 1 out]
        n155 = global read "Constants.vi" "DMA Elements Remaining"() -> (w405:string)
        n156 = call <vilib>:"NI VeriStand - Add Custom Device Channel.vi"("GUID (Default Channel)"=w405, "error in (no error)"=w407, "Channel"=w401, "Channel Name"=w404, "Parent Ref in"=w408) -> ("error out"=w409:errorcluster, "Parent Ref out"=w410:T3)  [unwired: 3 in, 2 out]
        n157 = global read "Constants.vi" "DMA Error"() -> (w402:string)
        n158 = call <vilib>:"NI VeriStand - Add Custom Device Channel.vi"("GUID (Default Channel)"=w402, "error in (no error)"=w409, "Channel"=w401, "Channel Name"=w403, "Parent Ref in"=w410) -> ("error out"=w406:errorcluster)  [unwired: 3 in, 3 out]
      }
    }
    n159 = Replace Array Subset(array=w30, new element=w21, index (row)=w23, index (col)=0 ("disabled index (col)")) -> (w29:string[][])
    n160 = call "Set Bitfile Object Name.vi"("error in (no error)"=w20, "Name"=w21, "Channel Ref"=w22) -> ("error out"=w19:errorcluster)  [unwired: 8 in]
  }
  n161 = call <vilib>:"NI VeriStand - Commit System Explorer Update Buffer.vi"("error in (no error)"=w6) -> ("error out"=w13:errorcluster)  [unwired: 10 in]
  n162 = property class="MCListbox (strict)"(reference=w4, error in=w13, "ItemNames"=w15) -> (error out=w12:errorcluster)  [unwired: 1 out]
  n163 = call "Enable Disable Add Remove buttons.vi"("not present item indexes"=w16, "error in (no error)"=w12, "selected items"=w3, "remove button"=w11, "add button"=w10) -> ("error out"=→"error out":errorcluster)  [unwired: 6 in]
  n164 = Bundle By Name(cluster="Listbox Refs in", "not present"=w16, "listbox text"=w15) -> (→"Listbox Refs out":T2)
